vi "OnOff Write.vi"(8 "error in":errorcluster, 10 "Value to Write":dbl, 11 "Power Supply In":refnum<class "Power Supply.lvclass">) -> (0 "error out":errorcluster, 1 "Changed or First Call?":bool, 2 "OnOff Out":bool, 3 "Power Supply Out":refnum<class "Power Supply.lvclass">)   [LabVIEW 2023, in "Power Supply.lvclass"]
uses:
  Power Supply.lvclass
  Power Supply.lvclass/Power Supply.ctl
  Low Level Capabilities/OnOff/OnOff.lvclass
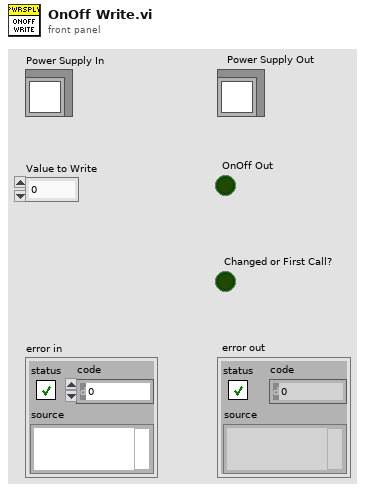
[diagram p1: front panel]
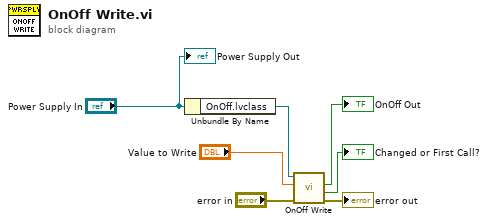
[diagram p0: block diagram]
diagram:
  n1 = Unbundle By Name("Power Supply In") -> ("OnOff.lvclass"=w1:refnum<class "OnOff.lvclass">)
  n2 = call-dynamic "OnOff Write.vi"("error in"="error in", "Value to Write"="Value to Write", "OnOff in"=w1) -> ("error out"=→"error out":errorcluster, "Changed or First Call?"=→"Changed or First Call?":bool, "OnOff Out"=→"OnOff Out":bool)  [unwired: 5 in, 1 out]
  "Power Supply Out" <- "Power Supply In"
